vi "conversionConfigGraphNum.vi"(1 "Config":T1={"action"=enum."PIV", "nb_periodes"=0, "t_periode"=1, "nb_pulse_prechauffe"=0, "nb_skip_frame_PIV"=0, "nb_skip_frame_LAT"=0, "t_FL1_start"=0, "t_FL1_stop"=0, "t_QS1_start"=0, "t_QS1_stop"=0, "t_FL2_start"=0, "t_FL2_stop"=0, "t_QS2_start"=0, "t_QS2_stop"=0, "t_LAT_start"=0, "t_LAT_stop"=0, "t_FRAME1_start"=0, "t_FRAME1_stop"=0, "t_FRAME2_start"=0, "t_FRAME2_stop"=0}) -> (0 "digital waveform":digitalwaveform(waveform)={"t0"=timestamp(0 s since 1904-01-01), "dt"=0.0, "Y"={"transitions"=[], "data"=[]}, "error"={"status"=FALSE, "code"=37421928, "source"=""}})   [LabVIEW 2020]
uses:
  configFPGA.ctl
  <vilib>/Waveform/DWDTOps.llb/DWDT Boolean Array to Digital.vi
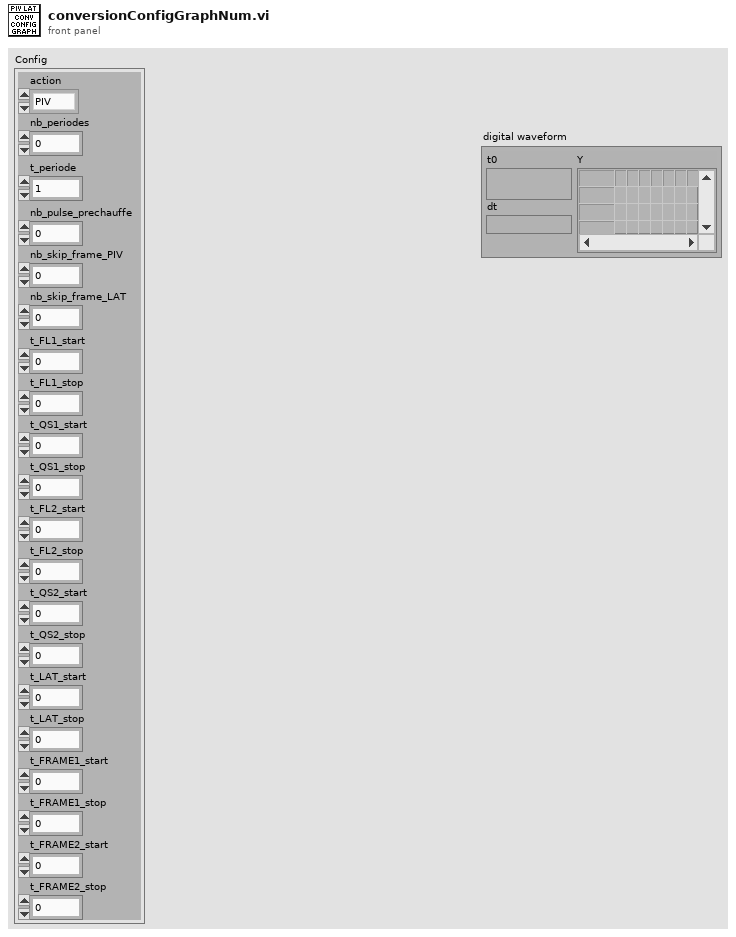
[diagram p1: front panel]
types:
  T1 = typedef "configFPGA.ctl" = cluster{"action":enum8{"PIV", "PIV + LAT", "STOP"}, "nb_periodes":u16, "t_periode":u32, "nb_pulse_prechauffe":u8, "nb_skip_frame_PIV":u8, "nb_skip_frame_LAT":u8, "t_FL1_start":u32, "t_FL1_stop":u32, "t_QS1_start":u32, "t_QS1_stop":u32, "t_FL2_start":u32, "t_FL2_stop":u32, "t_QS2_start":u32, "t_QS2_stop":u32, "t_LAT_start":u32, "t_LAT_stop":u32, "t_FRAME1_start":u32, "t_FRAME1_stop":u32, "t_FRAME2_start":u32, "t_FRAME2_stop":u32}
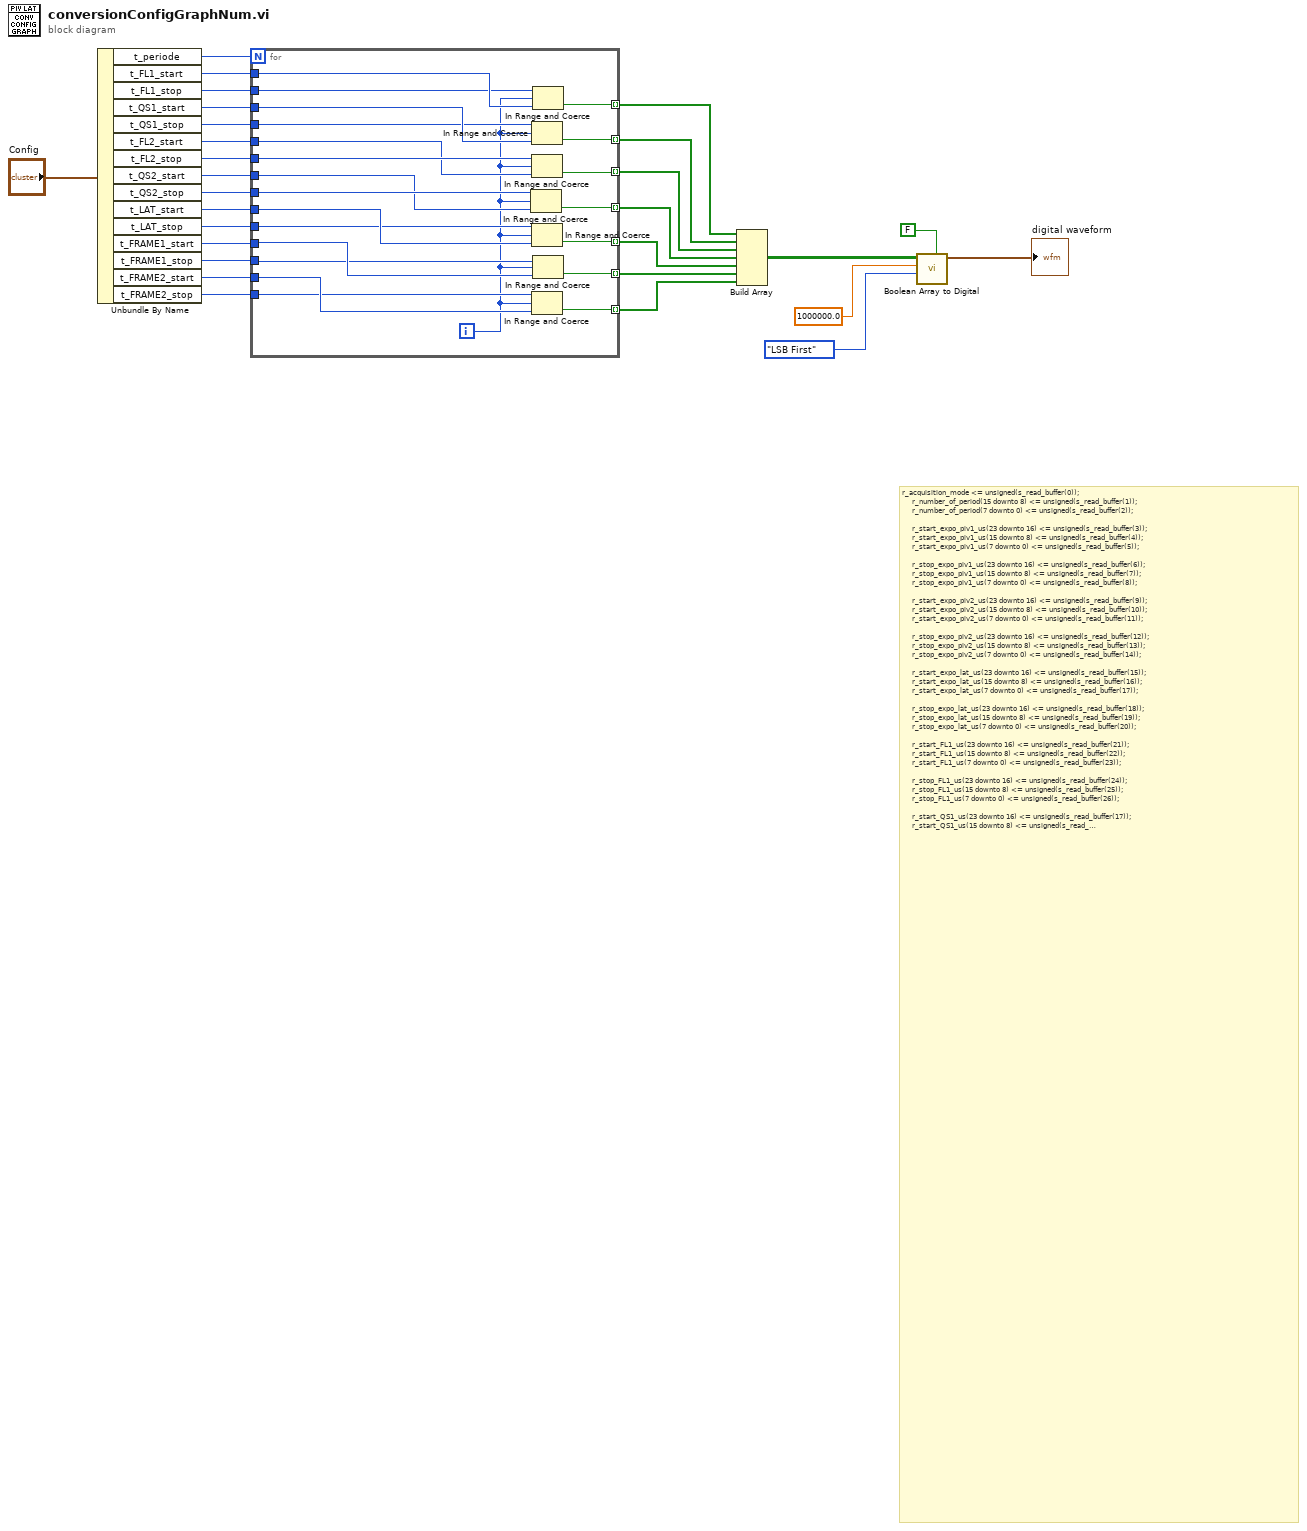
[diagram p0: block diagram]
diagram:
  # "r_acquisition_mode <= unsigned(s_read_buffer(0));\n     r_number_of_period(15 downto 8) <= unsigned(s_read_buffer(1));\n\t\t\t\t\tr_number_of_period(7 downto 0) <= unsigned(s_read_buffer(2));\n\t\t\t\t\t\n\t\t\t\t\tr_start_expo_piv1_us(23 downto 16) <= unsigned(s_read_buffer(3));\n\t\t\t\t\tr_start_expo_piv1_us(15 downto 8) <= unsigned(s_read_buffer(4));\n\t\t\t\t\tr_start_expo_piv1_us(7 downto 0) <= unsigned(s_read_buffer(5));\n\t\t\t\t\t\n\t\t\t\t\tr_stop_expo_piv1_us(23 downto 16) <= unsigned(s_read_buffer(6));\n\t\t\t\t\tr_stop_expo_piv1_us(15 downto 8) <= unsigned(s_read_buffer(7));\n\t\t\t\t\tr_stop_expo_piv1_us(7 downto 0) <= unsigned(s_read_buffer(8));\n\t\t\t\t\t\n\t\t\t\t\tr_start_expo_piv2_us(23 downto 16) <= unsigned(s_read_buffer(9));\n\t\t\t\t\tr_start_expo_piv2_us(15 downto 8) <= unsigned(s_read_buffer(10));\n\t\t\t\t\tr_start_expo_piv2_us(7 downto 0) <= unsigned(s_read_buffer(11));\n\t\t\t\t\t\n\t\t\t\t\tr_stop_expo_piv2_us(23 downto 16) <= unsigned(s_read_buffer(12));\n\t\t\t\t\tr_stop_expo_piv2_us(15 downto 8) <= unsigned(s_read_buffer(13));\n\t\t\t\t\tr_stop_expo_piv2_us(7 downto 0) <= unsigned(s_read_buffer(14));\n\t\t\t\t\t\n\t\t\t\t\tr_start_expo_lat_us(23 downto 16) <= unsigned(s_read_buffer(15));\n\t\t\t\t\tr_start_expo_lat_us(15 downto 8) <= unsigned(s_read_buffer(16));\n\t\t\t\t\tr_start_expo_lat_us(7 downto 0) <= unsigned(s_read_buffer(17));\n\t\t\t\t\t\n\t\t\t\t\tr_stop_expo_lat_us(23 downto 16) <= unsigned(s_read_buffer(18));\n\t\t\t\t\tr_stop_expo_lat_us(15 downto 8) <= unsigned(s_read_buffer(19));\n\t\t\t\t\tr_stop_expo_lat_us(7 downto 0) <= unsigned(s_read_buffer(20));\n\t\t\t\t\t\n\t\t\t\t\tr_start_FL1_us(23 downto 16) <= unsigned(s_read_buffer(21));\n\t\t\t\t\tr_start_FL1_us(15 downto 8) <= unsigned(s_read_buffer(22));\n\t\t\t\t\tr_start_FL1_us(7 downto 0) <= unsigned(s_read_buffer(23));\n\t\t\t\t\t\n\t\t\t\t\tr_stop_FL1_us(23 downto 16) <= unsigned(s_read_buffer(24));\n\t\t\t\t\tr_stop_FL1_us(15 downto 8) <= unsigned(s_read_buffer(25));\n\t\t\t\t\tr_stop_FL1_us(7 downto 0) <= unsigned(s_read_buffer(26));\n\t\t\t\t\t\n\t\t\t\t\tr_start_QS1_us(23 downto 16) <= unsigned(s_read_buffer(17));\n\t\t\t\t\tr_start_QS1_us(15 downto 8) <= unsigned(s_read_buffer(28));\n\t\t\t\t\tr_start_QS1_us(7 downto 0) <= unsigned(s_read_buffer(29));\n\t\t\t\t\t\n\t\t\t\t\tr_stop_QS1_us(23 downto 16) <= unsigned(s_read_buffer(30));\n\t\t\t\t\tr_stop_QS1_us(15 downto 8) <= unsigned(s_read_buffer(31));\n\t\t\t\t\tr_stop_QS1_us(7 downto 0) <= unsigned(s_read_buffer(32));\n\t\t\t\t\t\n\t\t\t\t\tr_start_FL2_us(23 downto 16) <= unsigned(s_read_buffer(33));\n\t\t\t\t\tr_start_FL2_us(15 downto 8) <= unsigned(s_read_buffer(34));\n\t\t\t\t\tr_start_FL2_us(7 downto 0) <= unsigned(s_read_buffer(35));\n\t\t\t\t\t\n\t\t\t\t\tr_stop_FL2_us(23 downto 16) <= unsigned(s_read_buffer(36));\n\t\t\t\t\tr_stop_FL2_us(15 downto 8) <= unsigned(s_read_buffer(37));\n\t\t\t\t\tr_stop_FL2_us(7 downto 0) <= unsigned(s_read_buffer(38));\n\t\t\t\t\t\n\t\t\t\t\tr_start_QS2_us(23 downto 16) <= unsigned(s_read_buffer(39));\n\t\t\t\t\tr_start_QS2_us(15 downto 8) <= unsigned(s_read_buffer(40));\n\t\t\t\t\tr_start_QS2_us(7 downto 0) <= unsigned(s_read_buffer(41));\n\t\t\t\t\t\n\t\t\t\t\tr_stop_QS2_us(23 downto 16) <= unsigned(s_read_buffer(42));\n\t\t\t\t\tr_stop_QS2_us(15 downto 8) <= unsigned(s_read_buffer(43));\n\t\t\t\t\tr_stop_QS2_us(7 downto 0) <= unsigned(s_read_buffer(44));\n\t\t\t\t\t\n\t\t\t\t\tw_i_period_us(23 downto 16) <= unsigned(s_read_buffer(45));\n\t\t\t\t\tw_i_period_us(15 downto 8) <= unsigned(s_read_buffer(46));\n\t\t\t\t\tw_i_period_us(7 downto 0) <= unsigned(s_read_buffer(47));\n\t\t\t\t\t\n\t\t\t\t\tr_number_pulse_heat_laser(7 downto 0) <= unsigned(s_read_buffer(48));\n\t\t\t\t\t\n\t\t\t\t\tr_PIV_skip_frames(7 downto 0) <= unsigned(s_read_buffer(49));\n\t\t\t\t\t\n\t\t\t\t\tr_LAT_skip_frames(7 downto 0) <= unsigned(s_read_buffer(50));"
  n1 = Unbundle By Name("Config") -> ("t_periode"=w27:u32, "t_FL1_start"=w26:u32, "t_FL1_stop"=w25:u32, "t_QS1_start"=w24:u32, "t_QS1_stop"=w23:u32, "t_FL2_start"=w22:u32, "t_FL2_stop"=w21:u32, "t_QS2_start"=w20:u32, "t_QS2_stop"=w19:u32, "t_LAT_start"=w18:u32, "t_LAT_stop"=w17:u32, "t_FRAME1_start"=w16:u32, "t_FRAME1_stop"=w15:u32, "t_FRAME2_start"=w14:u32, "t_FRAME2_stop"=w13:u32)
  n2 = for {
    N: w27 -> [_]
    tunnel: w26 -> [w50]
    tunnel: w25 -> [w49]
    tunnel: w24 -> [w48]
    tunnel: w23 -> [w47]
    tunnel: w22 -> [w43]
    tunnel: w21 -> [w44]
    tunnel: w20 -> [w45]
    tunnel: w19 -> [w46]
    tunnel: w18 -> [w42]
    tunnel: w17 -> [w41]
    tunnel: w16 -> [w40]
    tunnel: w15 -> [w39]
    tunnel: w14 -> [w38]
    tunnel: w13 -> [w37]
    tunnel: [w35] -> w12 mode=indexing
    tunnel: [w34] -> w11 mode=indexing
    tunnel: [w33] -> w10 mode=indexing
    tunnel: [w32] -> w9 mode=indexing
    tunnel: [w31] -> w8 mode=indexing
    tunnel: [w30] -> w7 mode=indexing
    tunnel: [w29] -> w6 mode=indexing
    i -> [w36]
    n3 = In Range and Coerce(upper limit=w46, x=w36, lower limit=w45) -> (In Range?=w32:bool)  [unwired: 1 out]
    n4 = In Range and Coerce(upper limit=w47, x=w36, lower limit=w48) -> (In Range?=w34:bool)  [unwired: 1 out]
    n5 = In Range and Coerce(upper limit=w44, x=w36, lower limit=w43) -> (In Range?=w33:bool)  [unwired: 1 out]
    n6 = In Range and Coerce(upper limit=w41, x=w36, lower limit=w42) -> (In Range?=w31:bool)  [unwired: 1 out]
    n7 = In Range and Coerce(upper limit=w37, x=w36, lower limit=w38) -> (In Range?=w29:bool)  [unwired: 1 out]
    n8 = In Range and Coerce(upper limit=w49, x=w36, lower limit=w50) -> (In Range?=w35:bool)  [unwired: 1 out]
    n9 = In Range and Coerce(upper limit=w39, x=w36, lower limit=w40) -> (In Range?=w30:bool)  [unwired: 1 out]
  }
  n10 = Build Array(w12, w11, w10, w9, w8, w7, w6) -> (w2:bool[][])
  n11 = call-poly <vilib>:"Boolean Array to Digital.vi"("compress data (F)"=FALSE, "mode"=enum16{"LSB First", "MSB First"}."LSB First", "sample rate"=1000000.0, "boolean array"=w2) -> ("digital waveform"=→"digital waveform":digitalwaveform)  [unwired: 6 in, 1 out]
